vi "getAllEvents.vi"(8 "error in (no error)":errorcluster, 11 "ScriptEventList in":refnum<class "ScriptEventList.lvclass">) -> (0 "error out":errorcluster, 1 "allStrings":string[][](array[string]), 2 "allScriptEvents":refnum<class "ScriptEvent.lvclass">[](array[class]), 3 "ScriptEventList out":refnum<class "ScriptEventList.lvclass">)   [LabVIEW 2011, in "Tools.lvlib" / "Scripting.lvlib" / "ScriptEventList.lvclass"]
uses:
  ScriptEventList.lvclass
  ScriptEvent.lvclass
  ScriptEventList.lvclass/ScriptEventList.ctl
  ScriptEvents/Ramp/RampEvent/RampEvent.lvclass
  ScriptEvents/SingleTone/SingleTone.lvclass
  ScriptEvents/Rf Event/rf.lvclass
  ScriptEvents/RfRamp/RfRamp.lvclass
  ScriptEvents/SingleTone/SingleToneRamp/SingleToneRamp.lvclass
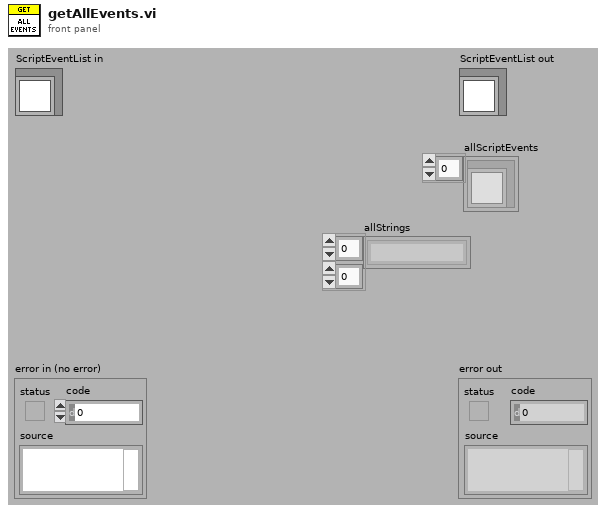
[diagram p1: front panel]
types:
  T1 = enum16{"changeValue", "pulse", "clock", "rampUp", "rampDown", "singleTone", "singleToneRamp", "playFile", "rf", "rfRamp", "delay"}
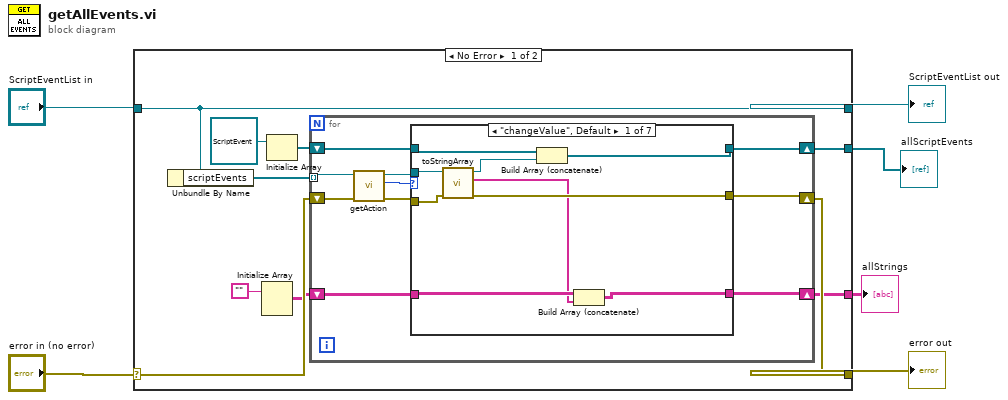
[diagram p0: block diagram]
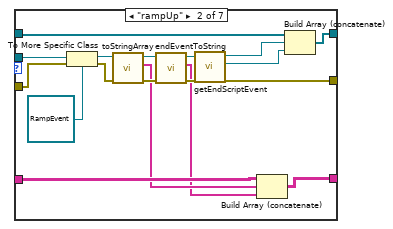
[diagram p2: hidden frame]
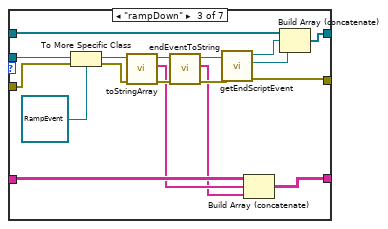
[diagram p3: hidden frame]
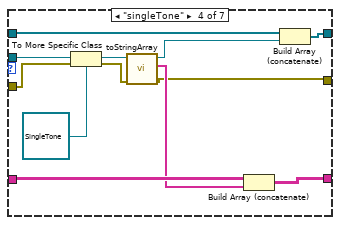
[diagram p4: hidden frame]
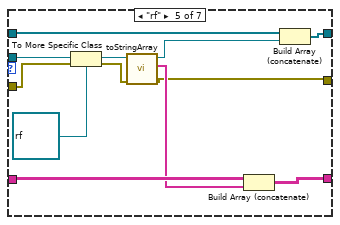
[diagram p5: hidden frame]
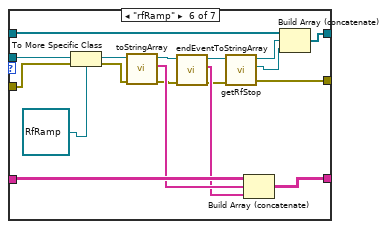
[diagram p6: hidden frame]
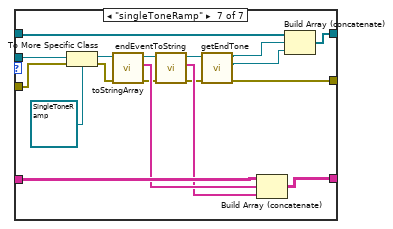
[diagram p7: hidden frame]
diagram:
  n1 = case shown="No Error" "error in (no error)" {
    selector: "error in (no error)" -> [w9 w133]
    tunnel: [w11 w133] -> w5
    tunnel: [w16 w132] -> w3
    tunnel: "ScriptEventList in" -> [w16 w132]
    tunnel: [w12 _] -> w2
    tunnel: [w7 _] -> w1
    frame No Error {
      n2 = Unbundle By Name(w16) -> ("scriptEvents"=w15:refnum<class "ScriptEvent.lvclass">[])
      n3 = Initialize Array("") -> (w8:string[][])  [unwired: 2 in]
      n4 = Initialize Array(refnum<class "ScriptEvent.lvclass"> refnum ("Tools.lvlib:Scripting.lvlib:ScriptEvent.lvclass")) -> (w13:refnum<class "ScriptEvent.lvclass">[])  [unwired: 1 in]
      n5 = for {
        tunnel: w15 -> [w26] mode=indexing
        shift-right: [w24] -> w12
        shift-left: w13 -> [w19]
        shift-right: [w20] -> w11
        shift-left: w9 -> [w21]
        shift-right: [w17] -> w7
        shift-left: w8 -> [w18]
        n6 = call "getAction.vi"("error in (no error)"=w21, "ScriptEvent.lvclass in"=w26) -> ("error out"=w22:errorcluster, "action"=w25:T1, "ScriptEvent.lvclass out"=w23:refnum<class "ScriptEvent.lvclass">)  [unwired: 7 in]
        n7 = case shown="\"changeValue\", Default" w25 {
          tunnel: w19 -> [w35 w50 w68 w81 w93 w111 w129]
          tunnel: [w34 w49 w67 w80 w92 w110 w128] -> w24
          tunnel: w23 -> [w33 w52 w70 w83 w95 w113 w131]
          tunnel: w22 -> [w32 w51 w69 w82 w94 w112 w130]
          tunnel: [w30 w46 w64 w72 w85 w96 w114] -> w20
          tunnel: w18 -> [w29 w39 w57 w77 w89 w107 w125]
          tunnel: [w28 w36 w56 w76 w88 w106 w123] -> w17
          frame "changeValue", Default {
            n8 = call-dynamic "toStringArray.vi"("error in (no error)"=w32, "ScriptEvent in"=w33) -> ("error out"=w30:errorcluster, "eventStringArray"=w27:string[], "ScriptEvent out"=w31:refnum<class "ScriptEvent.lvclass">)  [unwired: 7 in]
            n9 = Build Array (concatenate)(w35, w31) -> (w34:refnum<class "ScriptEvent.lvclass">[])
            n10 = Build Array (concatenate)(w29, w27) -> (w28:string[][])
          }
          frame "rampUp" {
            n11 = To More Specific Class(target class=refnum<class "RampEvent.lvclass"> refnum ("Tools.lvlib:Scripting.lvlib:RampEvent.lvclass"), reference=w52, error in=w51) -> (specific class reference=w45:refnum<class "RampEvent.lvclass">, error out=w44:errorcluster)
            n12 = call-dynamic "toStringArray.vi"("error in (no error)"=w44, "RampEvent in"=w45) -> ("error out"=w43:errorcluster, "eventStringArray"=w38:string[], "RampEvent out"=w42:refnum<class "RampEvent.lvclass">)  [unwired: 7 in]
            n13 = call "endEventToString.vi"("error in (no error)"=w43, "RampEvent in"=w42) -> ("error out"=w40:errorcluster, "eventStringArray"=w37:string[], "RampEvent out"=w41:refnum<class "RampEvent.lvclass">)  [unwired: 7 in]
            n14 = call "getEndScriptEvent.vi"("error in (no error)"=w40, "RampEvent.lvclass in"=w41) -> ("error out"=w46:errorcluster, "ScriptEvent.lvclass"=w47:refnum<class "ScriptEvent.lvclass">, "RampEvent.lvclass out"=w48:refnum<class "RampEvent.lvclass">)  [unwired: 7 in]
            n15 = Build Array (concatenate)(w39, w38, w37) -> (w36:string[][])
            n16 = Build Array (concatenate)(w50, w48, w47) -> (w49:refnum<class "ScriptEvent.lvclass">[])
          }
          frame "rampDown" {
            n17 = To More Specific Class(target class=refnum<class "RampEvent.lvclass"> refnum ("Tools.lvlib:Scripting.lvlib:RampEvent.lvclass"), reference=w70, error in=w69) -> (specific class reference=w60:refnum<class "RampEvent.lvclass">, error out=w59:errorcluster)
            n18 = call-dynamic "toStringArray.vi"("error in (no error)"=w59, "RampEvent in"=w60) -> ("error out"=w58:errorcluster, "eventStringArray"=w55:string[], "RampEvent out"=w61:refnum<class "RampEvent.lvclass">)  [unwired: 7 in]
            n19 = call "endEventToString.vi"("error in (no error)"=w58, "RampEvent in"=w61) -> ("error out"=w63:errorcluster, "eventStringArray"=w54:string[], "RampEvent out"=w62:refnum<class "RampEvent.lvclass">)  [unwired: 7 in]
            n20 = call "getEndScriptEvent.vi"("error in (no error)"=w63, "RampEvent.lvclass in"=w62) -> ("error out"=w64:errorcluster, "ScriptEvent.lvclass"=w65:refnum<class "ScriptEvent.lvclass">, "RampEvent.lvclass out"=w66:refnum<class "RampEvent.lvclass">)  [unwired: 7 in]
            n21 = Build Array (concatenate)(w57, w55, w54) -> (w56:string[][])
            n22 = Build Array (concatenate)(w68, w66, w65) -> (w67:refnum<class "ScriptEvent.lvclass">[])
          }
          frame "singleTone" {
            n23 = To More Specific Class(target class=refnum<class "SingleTone.lvclass"> refnum ("Tools.lvlib:Scripting.lvlib:SingleTone.lvclass"), reference=w83, error in=w82) -> (specific class reference=w79:refnum<class "SingleTone.lvclass">, error out=w78:errorcluster)
            n24 = call-dynamic "toStringArray.vi"("error in (no error)"=w78, "SingleTone in"=w79) -> ("error out"=w72:errorcluster, "eventStringArray"=w75:string[], "SingleTone out"=w73:refnum<class "SingleTone.lvclass">)  [unwired: 7 in]
            n25 = Build Array (concatenate)(w77, w75) -> (w76:string[][])
            n26 = Build Array (concatenate)(w81, w73) -> (w80:refnum<class "ScriptEvent.lvclass">[])
          }
          frame "rf" {
            n27 = To More Specific Class(target class=refnum<class "rf.lvclass"> refnum ("Tools.lvlib:Scripting.lvlib:rf.lvclass"), reference=w95, error in=w94) -> (specific class reference=w91:refnum<class "rf.lvclass">, error out=w90:errorcluster)
            n28 = call-dynamic "toStringArray.vi"("error in (no error)"=w90, "rf in"=w91) -> ("error out"=w85:errorcluster, "eventStringArray"=w87:string[], "rf out"=w86:refnum<class "rf.lvclass">)  [unwired: 7 in]
            n29 = Build Array (concatenate)(w89, w87) -> (w88:string[][])
            n30 = Build Array (concatenate)(w93, w86) -> (w92:refnum<class "ScriptEvent.lvclass">[])
          }
          frame "rfRamp" {
            n31 = To More Specific Class(target class=refnum<class "RfRamp.lvclass"> refnum ("Tools.lvlib:Scripting.lvlib:RfRamp.lvclass"), reference=w113, error in=w112) -> (specific class reference=w109:refnum<class "RfRamp.lvclass">, error out=w108:errorcluster)
            n32 = call-dynamic "toStringArray.vi"("error in (no error)"=w108, "RfRamp in"=w109) -> ("error out"=w102:errorcluster, "eventStringArray"=w105:string[], "RfRamp out"=w103:refnum<class "RfRamp.lvclass">)  [unwired: 7 in]
            n33 = call "endEventToStringArray.vi"("error in (no error)"=w102, "RfRamp in"=w103) -> ("error out"=w99:errorcluster, "eventStringArray"=w101:string[], "RfRamp out"=w100:refnum<class "RfRamp.lvclass">)  [unwired: 7 in]
            n34 = call "getRfStop.vi"("error in (no error)"=w99, "RfRamp in"=w100) -> ("error out"=w96:errorcluster, "rfStop"=w97:refnum<class "rf.lvclass">, "RfRamp out"=w98:refnum<class "RfRamp.lvclass">)  [unwired: 7 in]
            n35 = Build Array (concatenate)(w107, w105, w101) -> (w106:string[][])
            n36 = Build Array (concatenate)(w111, w98, w97) -> (w110:refnum<class "ScriptEvent.lvclass">[])
          }
          frame "singleToneRamp" {
            n37 = To More Specific Class(target class=refnum<class "SingleToneRamp.lvclass"> refnum ("Tools.lvlib:Scripting.lvlib:SingleToneRamp.lvclass"), reference=w131, error in=w130) -> (specific class reference=w127:refnum<class "SingleToneRamp.lvclass">, error out=w126:errorcluster)
            n38 = call-dynamic "toStringArray.vi"("error in (no error)"=w126, "SingleToneRamp in"=w127) -> ("error out"=w121:errorcluster, "eventStringArray"=w124:string[], "SingleToneRamp out"=w120:refnum<class "SingleToneRamp.lvclass">)  [unwired: 7 in]
            n39 = call "endEventToString.vi"("error in (no error)"=w121, "SingleToneRamp in"=w120) -> ("error out"=w118:errorcluster, "eventStringArray"=w119:string[], "SingleToneRamp out"=w117:refnum<class "SingleToneRamp.lvclass">)  [unwired: 7 in]
            n40 = call "getEndTone.vi"("error in (no error)"=w118, "SingleToneRamp.lvclass in"=w117) -> ("error out"=w114:errorcluster, "endTone"=w115:refnum<class "SingleTone.lvclass">, "SingleToneRamp.lvclass out"=w116:refnum<class "SingleToneRamp.lvclass">)  [unwired: 7 in]
            n41 = Build Array (concatenate)(w125, w124, w119) -> (w123:string[][])
            n42 = Build Array (concatenate)(w129, w116, w115) -> (w128:refnum<class "ScriptEvent.lvclass">[])
          }
        }
      }
    }
    frame Error {
    }
  }
  "error out" <- w5
  "ScriptEventList out" <- w3
  "allScriptEvents" <- w2
  "allStrings" <- w1
